vi "subGenerateModulationParameters.vi"(9 "System Parameters":T2={"Symbol Rate"=8.0, "Symbols per Packet"=8, "Tx Oversample Factor"=0, "Rx Oversample Factor"=16, "Modulation Scheme"=enum."4-QAM", "filter length (symbols)"=8, "filter parameter"=0.5, "Training Sequence"=[], "Channel Length Estimate"=1, "Frequency Offset\nCorrection?"=TRUE} {"Symbol Rate" format="%#_6p"; "Training Sequence" format="%#_3p"; "filter parameter" format="%.2f"}, 11 "error in (no error)":errorcluster) -> (6 "Calculated Parameters":T1 {"matched filter coefficients" format="%.6g"; "pulse shaping filter coefficients" format="%.6g"}, 10 "System Parameters (out)":T2={"Symbol Rate"=8.0, "Symbols per Packet"=8, "Tx Oversample Factor"=0, "Rx Oversample Factor"=16, "Modulation Scheme"=enum."4-QAM", "filter length (symbols)"=8, "filter parameter"=0.5, "Training Sequence"=[], "Channel Length Estimate"=1, "Frequency Offset\nCorrection?"=TRUE} {"Symbol Rate" format="%#_6p"; "Training Sequence" format="%#_3p"; "filter parameter" format="%.2f"}, 15 "error out":errorcluster)   [LabVIEW 2011]
uses:
  ModulationParameters.ctl
  CalculatedParameters.ctl
  <vilib>/addons/Modulation/niDMT.lvlib
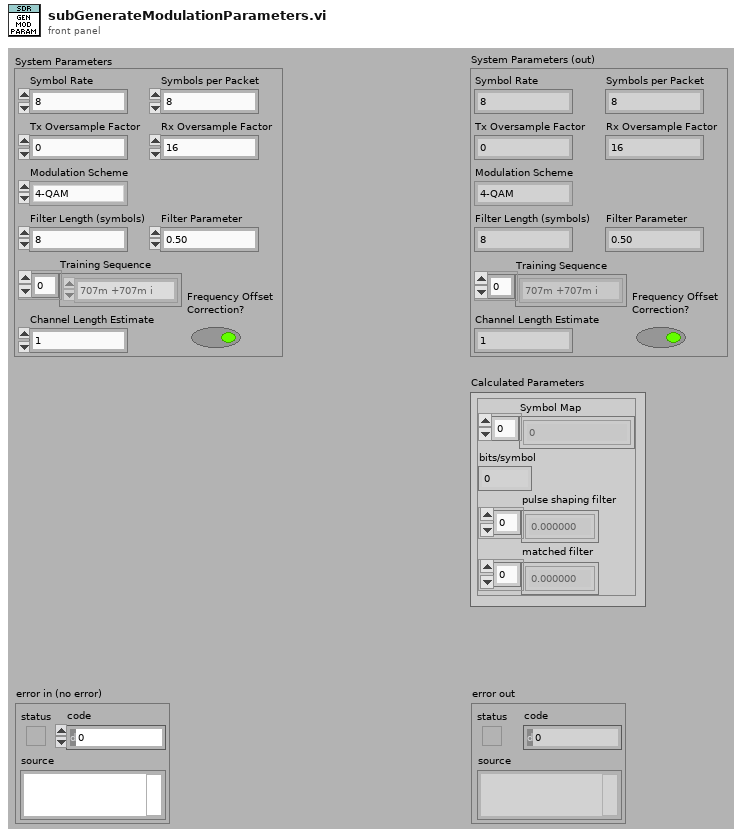
[diagram p1: front panel]
types:
  T1 = typedef "CalculatedParameters.ctl" = cluster{"Symbol Map":cdb[], "bits/symbol":i32, "pulse shaping filter coefficients":dbl[], "matched filter coefficients":dbl[]}
  T2 = typedef "ModulationParameters.ctl" = cluster{"Symbol Rate":dbl, "Symbols per Packet":i32, "Tx Oversample Factor":i32, "Rx Oversample Factor":i32, "Modulation Scheme":enum16{"4-QAM", "16-QAM", "64-QAM"}, "filter length (symbols)":i32, "filter parameter":dbl, "Training Sequence":cdb[], "Channel Length Estimate":i32, "Frequency Offset\nCorrection?":bool}
  T3 = enum16{"FSK", "PSK", "QAM", "MSK", "PAM", "ASK", "CPM"}
  T4 = enum16{"none", "Raised Cosine", "Root Raised Cos", "Gaussian"}
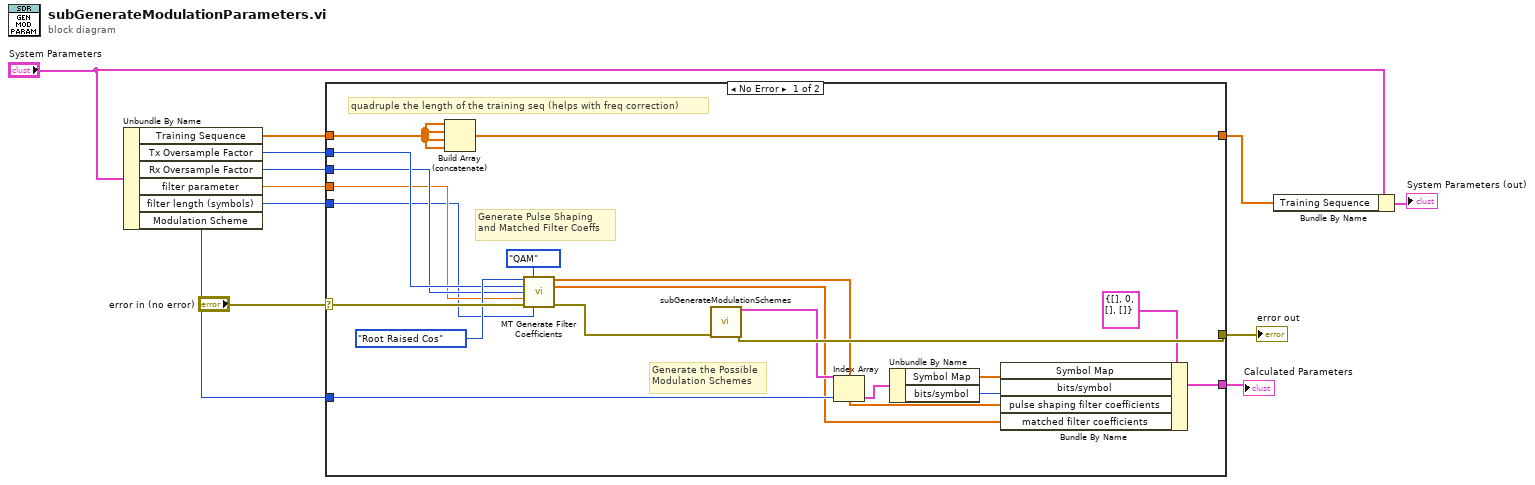
[diagram p0: block diagram]
diagram:
  n1 = Unbundle By Name("System Parameters") -> ("Training Sequence"=w4:cdb[], "Tx Oversample Factor"=w5:i32, "Rx Oversample Factor"=w10:i32, "filter parameter"=w9:dbl, "filter length (symbols)"=w8:i32, "Modulation Scheme"=w3:enum16{"4-QAM", "16-QAM", "64-QAM"})
  n2 = case shown="No Error" "error in (no error)" {
    selector: "error in (no error)" -> [w32 w34]
    tunnel: [w29 w34] -> w11
    tunnel: w5 -> [w28 _]
    tunnel: w10 -> [w27 _]
    tunnel: w9 -> [w26 _]
    tunnel: w8 -> [w25 _]
    tunnel: w4 -> [w23 w33]
    tunnel: [w22 w33] -> w1
    tunnel: w3 -> [w20 _]
    tunnel: [w15 _] -> w2
    frame No Error {
      # "quadruple the length of the training seq (helps with freq correction)"
      # "Generate the Possible\nModulation Schemes"
      # "Generate Pulse Shaping\nand Matched Filter Coeffs"
      n3 = Build Array (concatenate)(w23, w23, w23, w23) -> (w22:cdb[])
      n4 = call <vilib>:"MT Generate Filter Coefficients.vi"("pulse shaping filter (none)"=T4."Root Raised Cos", "modulation type"=T3."QAM", "pulse shaping samples per symbol (16)"=w28, "matched samples per symbol (16)"=w27, "filter parameter"=w26, "error in (no error)"=w32, "filter length (symbols)"=w25) -> ("pulse shaping filter coefficients"=w14:dbl[], "matched filter coefficients"=w13:dbl[], "error out"=w24:errorcluster)  [unwired: 6 out]
      n5 = call "subGenerateModulationSchemes.vi"("error in (no error)"=w24) -> ("Modulation Schemes"=w21:cluster{"Symbol Map":cdb[], "bits/symbol":i32}[], "error out"=w29:errorcluster)  [unwired: 13 in]
      n6 = Index Array(array=w21, index=w20) -> (element=w19:cluster{"Symbol Map":cdb[], "bits/symbol":i32})
      n7 = Unbundle By Name(w19) -> ("Symbol Map"=w17:cdb[], "bits/symbol"=w16:i32)
      n8 = Bundle By Name(cluster=T1 {"Symbol Map"=[], "bits/symbol"=0, "pulse shaping filter coefficients"=[], "matched filter coefficients"=[]} ("Calculated Parameters"), "Symbol Map"=w17, "bits/symbol"=w16, "pulse shaping filter coefficients"=w14, "matched filter coefficients"=w13) -> (w15:T1)
    }
    frame Error {
    }
  }
  "error out" <- w11
  "Calculated Parameters" <- w2
  n9 = Bundle By Name(cluster="System Parameters", "Training Sequence"=w1) -> (→"System Parameters (out)":T2)
